vi "Register.vi"(6 "Get Last Broadcast Event (F)":bool, 7 "Event":refnum<class "Event.lvclass">, 8 "Error In":errorcluster, 9 "View Event Fire Handler":refnum<class "Abstract Event Message for View.lvclass">, 10 "Registrant Details":T1, 11 "Controller In":refnum<class "Controller.lvclass">) -> (0 "Error Out":errorcluster, 3 "Controller Out":refnum<class "Controller.lvclass">)   [LabVIEW 2023, in "MVC Actors.lvlib" / "Controller.lvclass"]
doc: "This method registers a specific Actors Enqueuer and a Zero Coupling based message (inheriting from Event Generated Msg.lvclass) to used when the specified Event is Fired anywhere inside the Event Source Actor."
uses:
  Controller.lvclass
  Event/Event.lvclass
  View Details.ctl
  <vilib>/ActorFramework/Message Enqueuer/Message Enqueuer.lvclass
  Event Handlers/Abstract Event Message for View/Abstract Event Message for View.lvclass
  Controller.lvclass/Controller.ctl
  Event Handler Details.ctl
  Event/Event.lvclass/Event.ctl
  <vilib>/Utility/error.llb/Error Cluster From Error Code.vi
  <vilib>/ErrorRing/Error Ring.xnode
  <resource>/AFDebug/AF Debug.lvlib
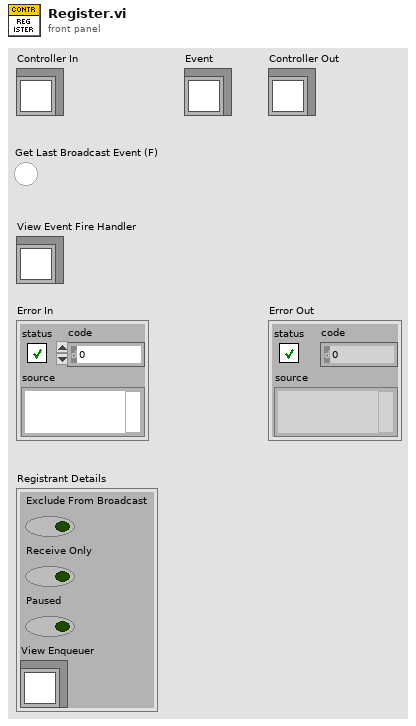
[diagram p1: front panel]
types:
  T1 = typedef "MVC Actors.lvlib/Controller.lvclass/View Details.ctl" = cluster{"Exclude From Broadcast":bool, "Receive Only":bool, "Paused":bool, "View Enqueuer":refnum<class "Message Enqueuer.lvclass">}
  T2 = typedef "MVC Actors.lvlib/Controller.lvclass/Event Handler Details.ctl" = cluster{"Exclude From Broadcast":bool, "Paused":bool, "View Event Fire Handler":refnum<class "Abstract Event Message for View.lvclass">}
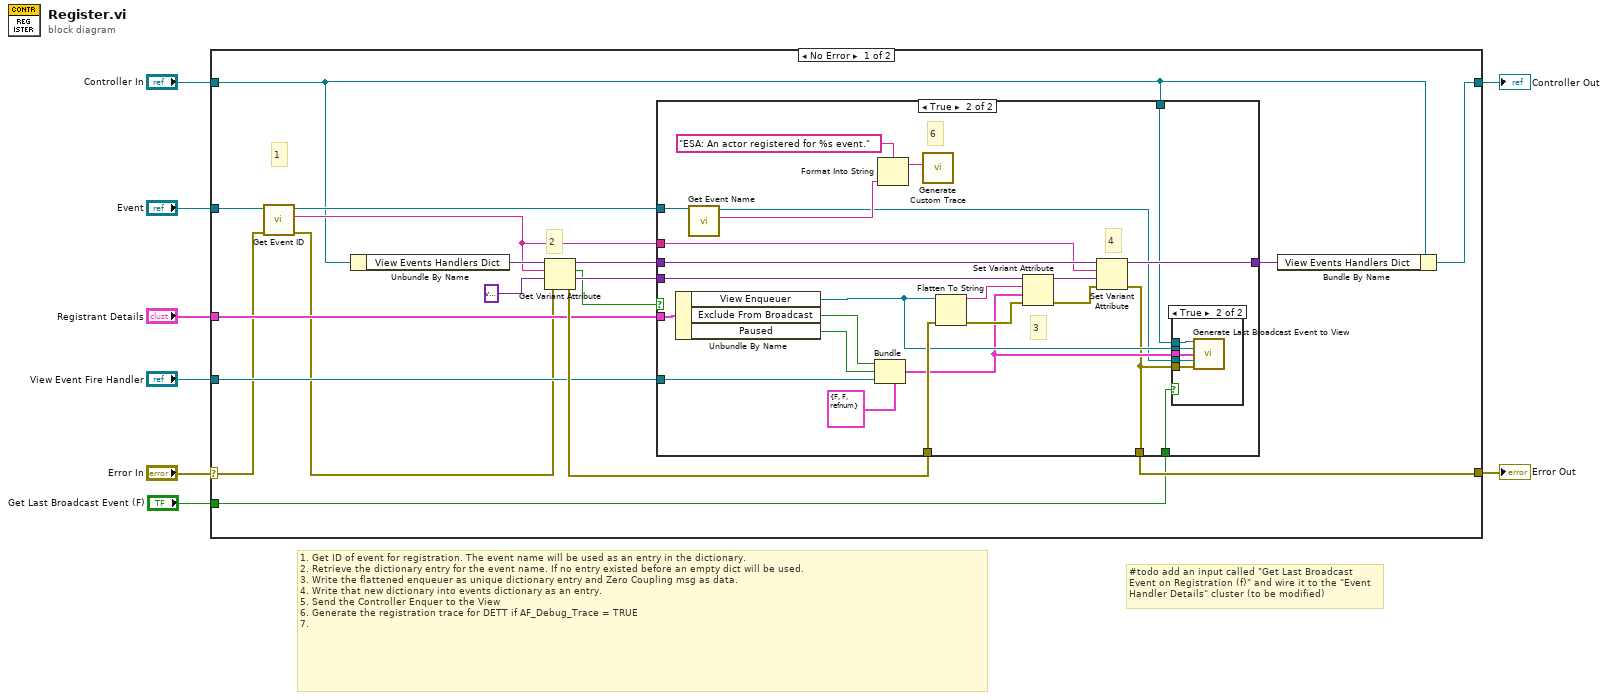
[diagram p0: block diagram]
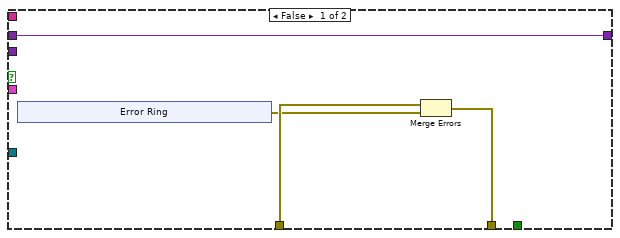
[diagram p2: hidden frame]
diagram:
  # "#todo add an input called \"Get Last Broadcast Event on Registration (f)\" and wire it to the \"Event Handler Details\" cluster (to be modified)"
  # "1. Get ID of event for registration. The event name will be used as an entry in the dictionary.\n2. Retrieve the dictionary entry for the event name. If no entry existed before an empty dict will be used.\n3. Write the flattened enqueuer as unique dictionary entry and Zero Coupling msg as data.\n4. Write that new dictionary into events dictionary as an entry.\n5. Send the Controller Enquer to the View\n6. Generate the registration trace for DETT if AF_Debug_Trace = TRUE\n7."
  n1 = case shown="No Error" "Error In" {
    selector: "Error In" -> [w15 w64]
    tunnel: "Controller In" -> [w9 w65]
    tunnel: "Event" -> [w16 _]
    tunnel: [w22 w65] -> w7
    tunnel: [w26 w64] -> w5
    tunnel: "Registrant Details" -> [w17 _]
    tunnel: "View Event Fire Handler" -> [w21 _]
    tunnel: "Get Last Broadcast Event (F)" -> [w10 _]
    frame No Error {
      # "2"
      # "1"
      n2 = call-dynamic "Get Event ID.vi"("error in (no error)"=w15, "Event in"=w16) -> ("error out"=w13:errorcluster, "Event ID"=w14:string, "Event out"=w11:refnum<class "Event.lvclass">)  [unwired: 7 in]
      n3 = Unbundle By Name(w9) -> ("View Events Handlers Dict"=w25:variant)
      n4 = Get Variant Attribute(Variant=w25, name=w14, default value (empty Variant)=variant ("variant"), error in=w13) -> (duplicate Variant=w24:variant, found=w12:bool, value=w19:variant, error out=w23:errorcluster)
      n5 = case shown="True" w12 {
        tunnel: [w29 w36] -> w26
        tunnel: w24 -> [w28 w58]
        tunnel: w23 -> [w30 w57]
        tunnel: w21 -> [_ w41]
        tunnel: [w28 w54] -> w20
        tunnel: w19 -> [_ w53]
        tunnel: w17 -> [_ w45]
        tunnel: w14 -> [_ w52]
        tunnel: w11 -> [_ w46]
        tunnel: w10 -> [_ w38]
        tunnel: w9 -> [_ w35]
        frame False {
          n6 = xnode "Error Ring"() -> ("error out"=w27:errorcluster)
          n7 = Merge Errors(w30, w27) -> (w29:errorcluster)
        }
        frame True {
          # "6"
          # "4"
          # "3"
          n8 = Unbundle By Name(w45) -> ("View Enqueuer"=w40:refnum<class "Message Enqueuer.lvclass">, "Exclude From Broadcast"=w43:bool, "Paused"=w42:bool)
          n9 = call "Get Event Name.vi"("Event In"=w46) -> ("Name"=w47:string, "Event Out"=w37:refnum<class "Event.lvclass">)  [unwired: 9 in]
          n10 = Bundle(cluster=T2 {"Exclude From Broadcast"=FALSE, "Paused"=FALSE, "View Event Fire Handler"=refnum} ("Sink Settings"), "Exclude From Broadcast"=w43, "Paused"=w42, "View Event Fire Handler"=w41) -> (w39:T2)
          n11 = Format Into String(format string="ESA: An actor registered for %s event." ("Custom Action"), w47) -> (resulting string=w48:string)  [unwired: 2 in, 1 out]
          n12 = call <resource>:"Generate Custom Trace.vi"("Custom Action"=w48) -> ()  [unwired: 11 in]
          n13 = Flatten To String(anything=w40, error in (no error)=w57) -> (data string=w56:string, error out=w51:errorcluster)  [unwired: 2 in, 1 out]
          n14 = Set Variant Attribute(Variant=w53, name=w56, value=w39, error in=w51) -> (Variant out=w55:variant, error out=w50:errorcluster)  [unwired: 1 out]
          n15 = Set Variant Attribute(Variant=w58, name=w52, value=w55, error in=w50) -> (Variant out=w54:variant, error out=w36:errorcluster)  [unwired: 1 out]
          n16 = case shown="True" w38 {
            tunnel: w40 -> [_ w63]
            tunnel: w39 -> [_ w62]
            tunnel: w37 -> [_ w61]
            tunnel: w36 -> [_ w60]
            tunnel: w35 -> [_ w59]
            frame False {
            }
            frame True {
              n17 = call "Generate Last Broadcast Event to View.vi"("Controller in"=w59, "View Enqueuer in"=w63, "Event Handler Details"=w62, "Event"=w61, "error in (no error)"=w60) -> ()  [unwired: 10 in, 1 out]
            }
          }
        }
      }
      n18 = Bundle By Name(cluster=w9, "View Events Handlers Dict"=w20) -> (w22:refnum<class "Controller.lvclass">)
    }
    frame Error {
    }
  }
  "Error Out" <- w5
  "Controller Out" <- w7
